vi "Results.Get.vi"(8 "error in (no error)":errorcluster, 11 "path":path) -> (0 "error out":errorcluster, 3 "Result":T1)   [LabVIEW 2015, in "Single Station Execution.lvlib"]
uses:
  Single Station Execution.lvlib
  Types/Results.Value.ctl
  NationalInstruments.VeriStand.ATMLTestResults
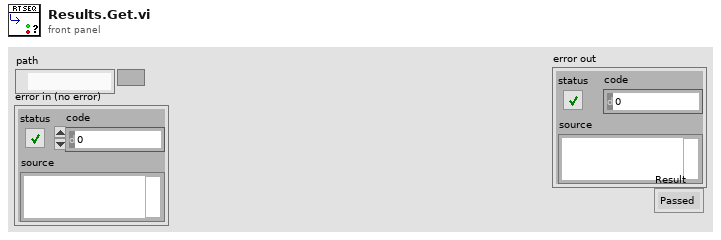
[diagram p1: front panel]
types:
  T1 = typedef "Single Station Execution.lvlib/Results.Value.ctl" = enum8{"Passed", "Failed", "Aborted"}
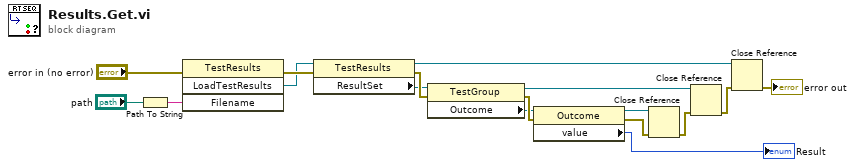
[diagram p0: block diagram]
diagram:
  n1 = Path To String(path="path") -> (string=w5:string)
  n2 = invoke class="TestResults" method="LoadTestResults"(error in="error in (no error)", "Filename"=w5) -> (error out=w17:errorcluster, "LoadTestResults"=w6:refnum<k24>)  [unwired: 2 in, 2 out]
  n3 = property class="TestResults"(reference=w6, error in=w17) -> (reference out=w7:refnum<k24>, error out=w16:errorcluster, "ResultSet"=w14:refnum<k24>)
  n4 = property class="TestGroup"(reference=w14, error in=w16) -> (reference out=w9:refnum<k24>, error out=w15:errorcluster, "Outcome"=w13:refnum<k24>)
  n5 = property class="Outcome"(reference=w13, error in=w15) -> (reference out=w12:refnum<k24>, error out=w11:errorcluster, "value"=→"Result":i32)
  n6 = Close Reference(reference=w12, error in (no error)=w11) -> (error out=w10:errorcluster)
  n7 = Close Reference(reference=w9, error in (no error)=w10) -> (error out=w8:errorcluster)
  n8 = Close Reference(reference=w7, error in (no error)=w8) -> (error out=→"error out":errorcluster)
